vi "Read Control cluster.vi"(8 "error in (no error)":errorcluster, 11 "Gage digitizer actor in":refnum<class "Gage digitizer actor.lvclass">) -> (0 "error out":errorcluster, 2 "Control cluster":T1={"Number of points"=816000.0, "Input Range"=10000, "Trigger Level"=29, "Trigger source"=TRUE} {"Trigger Level" min=-100 max=100 step=1 scale=-100.0..100.0; "Input Range" items=["+/- 5 V"=10000, "+/- 2 V"=4000, "+/- 1 V"=2000, "+/- 500 mV"=1000, "+/- 200 mV"=400, "+/- 100 mV"=200]; "Number of points" min=160.0 step=160.0}, 3 "Gage digitizer actor out":refnum<class "Gage digitizer actor.lvclass">)   [LabVIEW 2015, in "Gage digitizer actor.lvclass"]
uses:
  Gage digitizer actor.lvclass
  Basic controlls.ctl
  Gage digitizer actor.lvclass/Gage digitizer actor.ctl
panel:
  # "Basic Card Controlls"
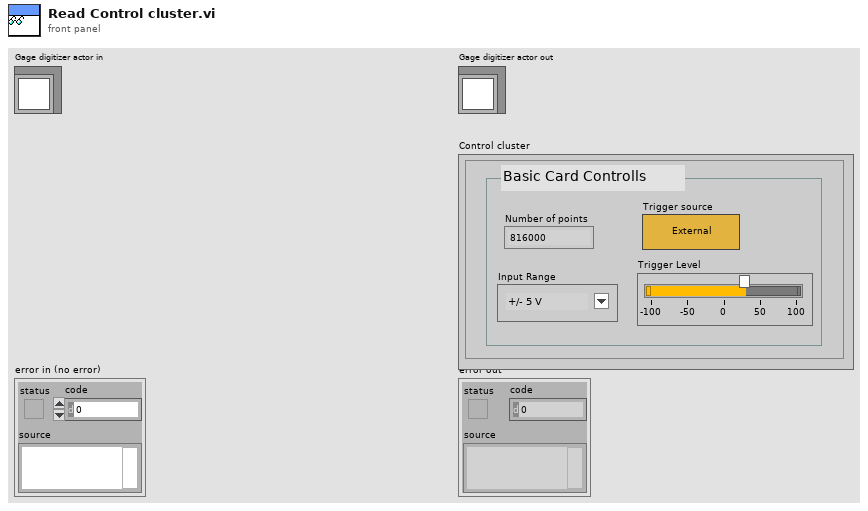
[diagram p1: front panel]
types:
  T1 = typedef "Basic controlls.ctl" = cluster{"Number of points":dbl, "Input Range":u32, "Trigger Level":i32, "Trigger source":bool}
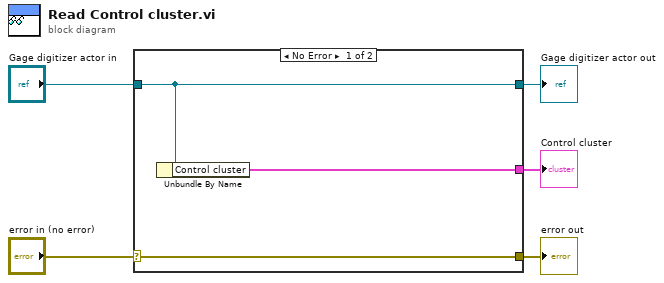
[diagram p0: block diagram]
diagram:
  n1 = case shown="No Error" "error in (no error)" {
    selector: "error in (no error)" -> [w8 w9]
    tunnel: [w8 w9] -> w4
    tunnel: [w7 w10] -> w2
    tunnel: "Gage digitizer actor in" -> [w7 w10]
    tunnel: [w6 _] -> w1
    frame No Error {
      n2 = Unbundle By Name(w7) -> ("Control cluster"=w6:T1)
    }
    frame Error {
    }
  }
  "error out" <- w4
  "Gage digitizer actor out" <- w2
  "Control cluster" <- w1
